vi "Neutral_1x48ch_to_2x24ch.vi"(8 "Error In":errorcluster, 11 "48ch_pb_array":T3 {"Label and Instructions"."Instruct Data" format="%#.2p"; "Label and Instructions"."Op Code" items=["Continue", "Stop", "Loop", "End Loop", "JSR", "RTS", "Go To", "Long Delay", "Wait"]; "Label and Instructions"."Time (s)" min=5e-08 format="%.2p"}) -> (0 "error out":errorcluster, 3 "1D_array_of_24ch_pb_array":cluster{"24ch_pb_array":T2}[](array[cluster]) {"24ch_pb_array"."Time (s)" min=5e-08 format="%.2p"; "24ch_pb_array"."Op Code" items=["Continue", "Stop", "Loop", "End Loop", "JSR", "RTS", "Go To", "Long Delay", "Wait"]; "24ch_pb_array"."Instruct Data" format="%#.2p"})   [LabVIEW 2016]
uses:
  Controls/PulseBlaster/48ch_pb_array.ctl
  Controls/PulseBlaster/48ch_single_timing_column_condensed.ctl
  Controls/PulseBlaster/24ch_pb_array.ctl
  Controls/PulseBlaster/24ch_single_timing_column.ctl
panel:
  in  "24ch_pb_array":T1[](array[typedef]) {"Time (s)" min=5e-08 format="%.2p"; "Op Code" items=["Continue", "Stop", "Loop", "End Loop", "JSR", "RTS", "Go To", "Long Delay", "Wait"]; "Instruct Data" format="%#.2p"}
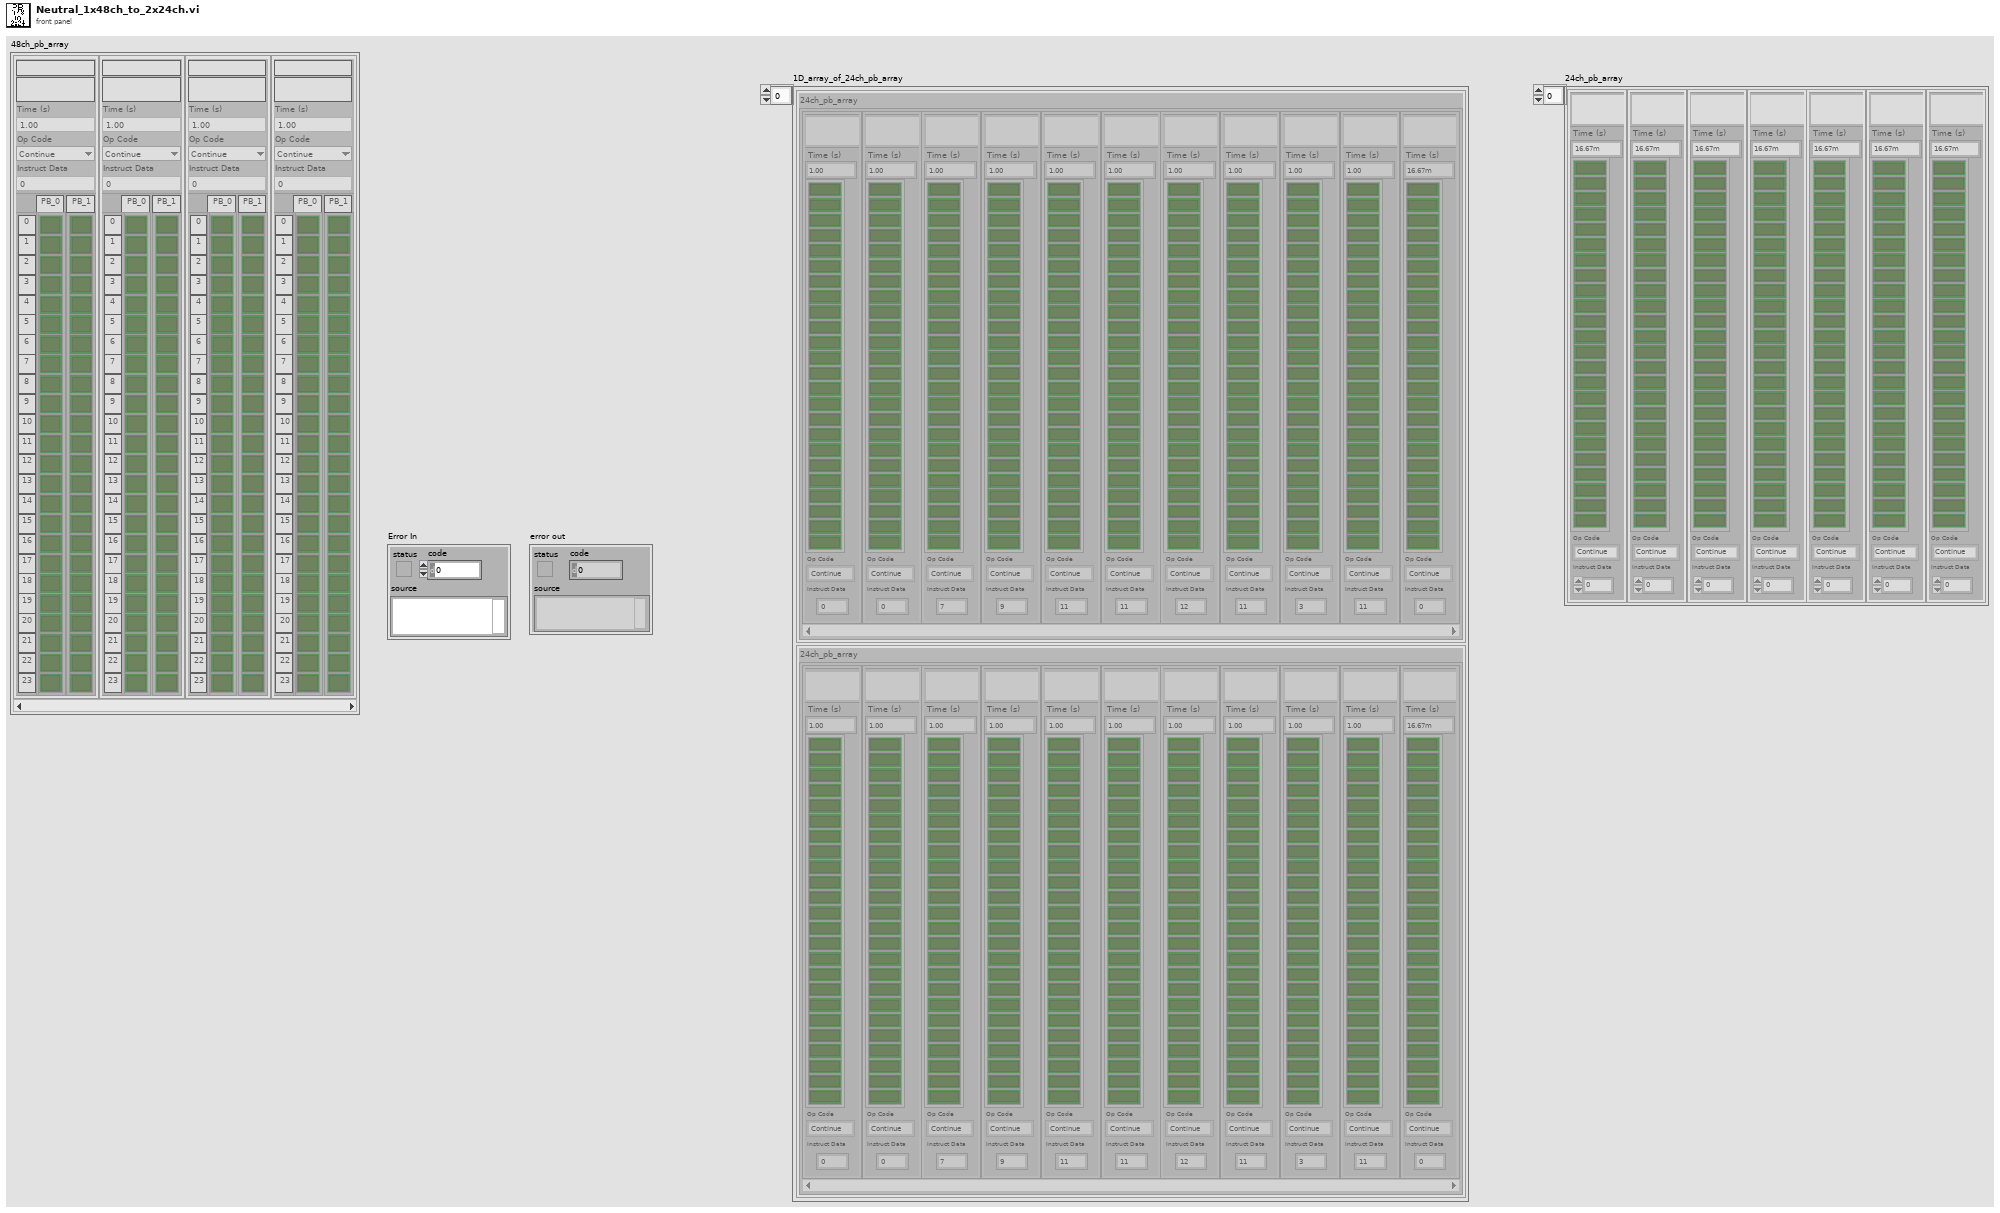
[diagram p1: front panel]
types:
  T1 = typedef "24ch_single_timing_column.ctl" = cluster{"Instruct Data":i32, "Op Code":i32, "Flags":bool[], "Comments":string, "Time (s)":dbl}
  T2 = typedef "24ch_pb_array.ctl" = T1[]
  T3 = typedef "48ch_pb_array.ctl" = T4[]
  T4 = typedef "48ch_single_timing_column_condensed.ctl" = cluster{"Label and Instructions":cluster{"Column Number":string, "Comments":string, "Time (s)        ":dbl, "Op Code":i32, "Instruct Data":i32}, "PB_1_Bools":bool[], "Column Number":string, "Column Number 2":string, "PB_0_Bools":bool[], "Ch_Labels":string[]}
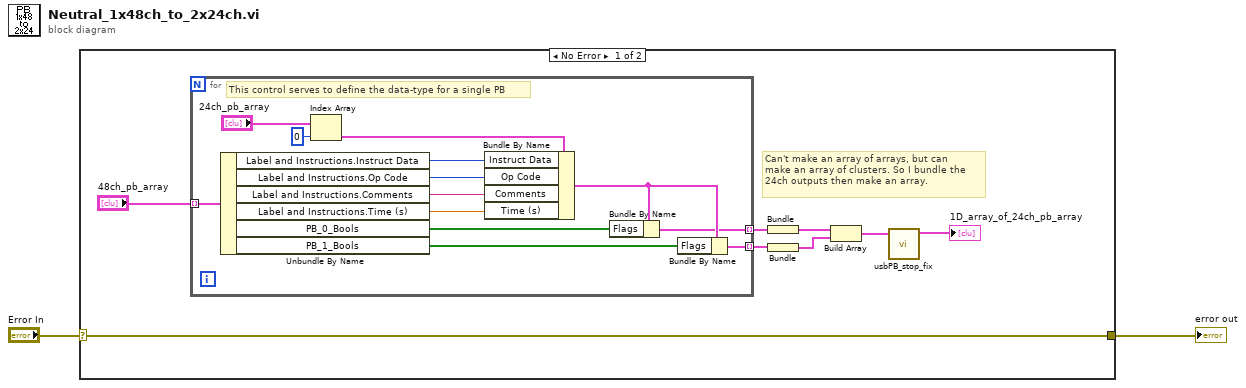
[diagram p0: block diagram]
diagram:
  n1 = case shown="No Error" "Error In" {
    selector: "Error In" -> [w9 w24]
    tunnel: [w9 w24] -> w1
    frame No Error {
      # "Can't make an array of arrays, but can\nmake an array of clusters. So I bundle the \n24ch outputs then make an array."
      n2 = for {
        tunnel: "48ch_pb_array" -> [w23] mode=indexing
        tunnel: [w15] -> w8 mode=indexing
        tunnel: [w14] -> w7 mode=indexing
        # "This control serves to define the data-type for a single PB"
        n3 = Unbundle By Name(w23) -> ("Label and Instructions.Instruct Data"=w22:i32, "Label and Instructions.Op Code"=w21:i32, "Label and Instructions.Comments"=w20:string, "Label and Instructions.Time (s)"=w19:dbl, "PB_0_Bools"=w18:bool[], "PB_1_Bools"=w16:bool[])
        n4 = Index Array(array="24ch_pb_array", index=0) -> (element=w11:T1)
        n5 = Bundle By Name(cluster=w11, "Instruct Data"=w22, "Op Code"=w21, "Comments"=w20, "Time (s)"=w19) -> (w17:T1)
        n6 = Bundle By Name(cluster=w17, "Flags"=w18) -> (w14:T1)
        n7 = Bundle By Name(cluster=w17, "Flags"=w16) -> (w15:T1)
      }
      n8 = Bundle(w7) -> (w6:cluster{T1[]})  [unwired: 1 in]
      n9 = Bundle(w8) -> (w5:cluster{T1[]})  [unwired: 1 in]
      n10 = Build Array(w6, w5) -> (w4:cluster{T1[]}[])
      n11 = call "usbPB_stop_fix.vi"("1D_array_of_24ch_pb_array\nIN"=w4) -> ("1D_array_of_24ch_pb_array\nOUT"=→"1D_array_of_24ch_pb_array":cluster{"24ch_pb_array":T2}[])  [unwired: 10 in]
    }
    frame Error {
    }
  }
  "error out" <- w1
